vi "Switch Matrix to Channel Array.vi"(7 "Card Slot #":u16=1 min=1 max=6, 10 "Switch Matrix":bool[][](array[boolean])) -> (2 "Channel Array":T1(array[cluster]))   [LabVIEW 2018, in "Keithley 3706.lvlib"]
uses:
  <instrlib>/Keithley 3706/Keithley 3706.lvlib
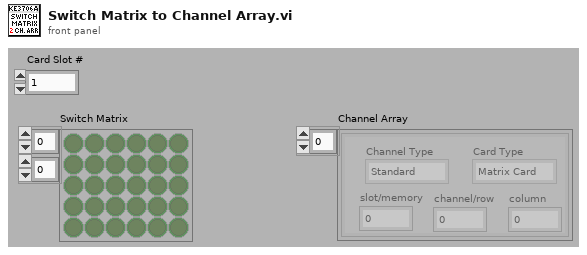
[diagram p1: front panel]
types:
  T1 = cluster{"slot/memory":i32, "channel/row":i32, "column":i32, "Channel Type":enum16{"Standard"}, "Card Type":enum16{"Matrix Card", "Multiplexer Card"}}[]
  T2 = cluster{"slot/memory":i32, "channel/row":i32, "column":i32, "Channel Type":enum16{"Standard"}, "Card Type":enum16{"Matrix Card", "Multiplexer Card"}}
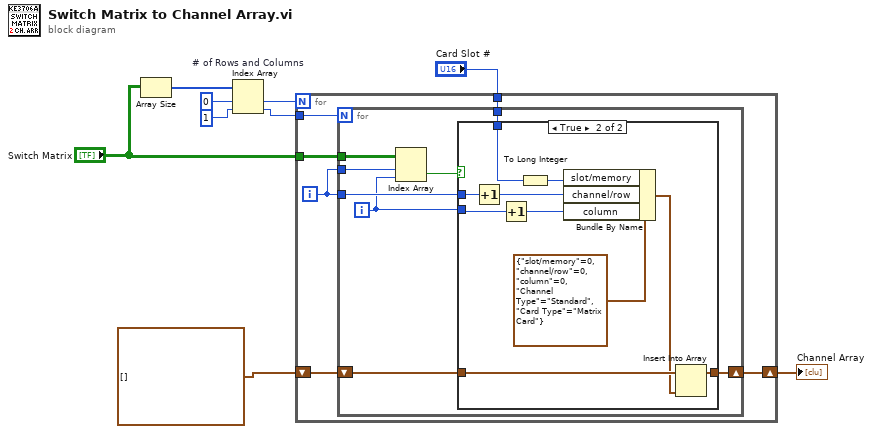
[diagram p0: block diagram]
diagram:
  n1 = Array Size(array="Switch Matrix") -> (size(s)=w6:i32[])
  n2 = Index Array "# of Rows and Columns"(array=w6, index #1=0 ("index"), index #2=1 ("index")) -> (element #1=w5:i32, element #2=w3:i32)
  n3 = for {
    N: w5 -> [_]
    tunnel: w3 -> [w15]
    tunnel: "Switch Matrix" -> [w14]
    tunnel: "Card Slot #" -> [w13]
    shift-right: [w10] -> w2
    shift-left: T1 [] -> [w11]
    i -> [w12]
    n4 = for {
      N: w15 -> [_]
      tunnel: w14 -> [w23]
      tunnel: w12 -> [w22]
      tunnel: w13 -> [w20]
      tunnel: w12 -> [w19]
      shift-right: [w16] -> w10
      shift-left: w11 -> [w17]
      i -> [w18]
      n5 = Index Array(array=w23, index (row)=w22, index (col)=w18) -> (element=w21:bool)
      n6 = case shown="True" w21 {
        tunnel: w20 -> [_ w25]
        tunnel: w19 -> [_ w30]
        tunnel: w18 -> [_ w31]
        tunnel: w17 -> [w24 w33]
        tunnel: [w24 w34] -> w16
        frame False {
        }
        frame True {
          n7 = Increment(x=w30) -> (x+1=w29:i32)
          n8 = Increment(x=w31) -> (x+1=w32:i32)
          n9 = To Long Integer(number=w25) -> (32bit integer=w26:i32)
          n10 = Bundle By Name(cluster=T2 {"slot/memory"=0, "channel/row"=0, "column"=0, "Channel Type"=enum."Standard", "Card Type"=enum."Matrix Card"} ("Channel Definition"), "slot/memory"=w26, "channel/row"=w29, "column"=w32) -> (w28:T2)
          n11 = Insert Into Array(array=w33, new element=w28) -> (w34:T1)  [unwired: 1 in]
        }
      }
    }
  }
  "Channel Array" <- w2
